vi "Update AppInst Ring.vi"(7 "OpenAppDialog":bool=TRUE, 8 "error in":errorcluster, 9 "Old Value":u16=65535, 10 "AppInst in":refnum<vi>, 11 "Ring in":refnum<vi>) -> (0 "error out":errorcluster, 1 "Selection Changed?":bool, 2 "AppInst out":refnum<vi>)   [LabVIEW 2013, in "LVTM.lvlib"]
uses:
  LVTM.lvlib
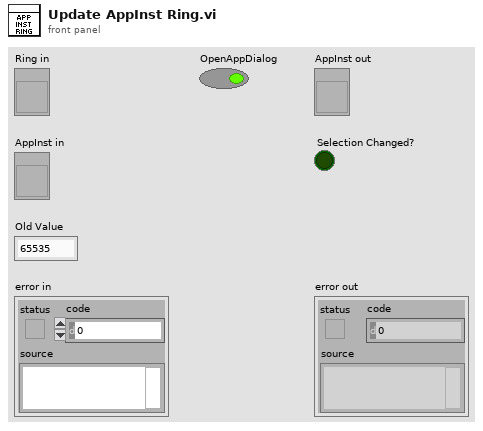
[diagram p1: front panel]
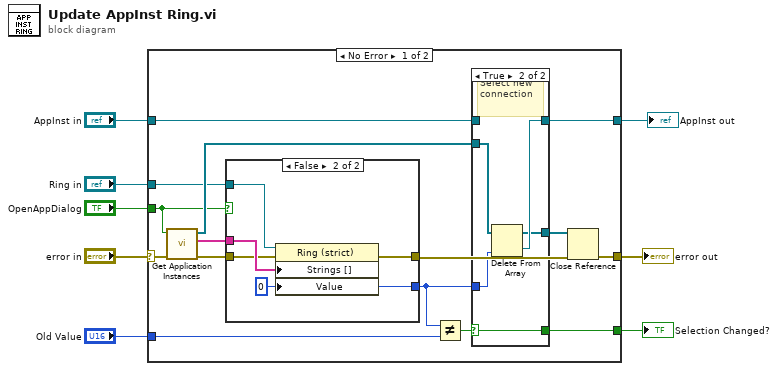
[diagram p0: block diagram]
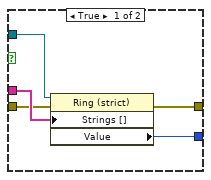
[diagram p2: hidden frame]
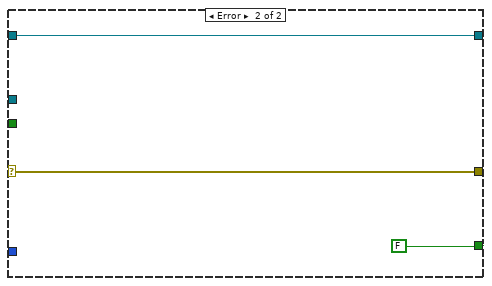
[diagram p4: hidden frame]
diagram:
  n1 = case shown="No Error" "error in" {
    selector: "error in" -> [w19 w44]
    tunnel: "Ring in" -> [w16 _]
    tunnel: [w22 w42] -> w7
    tunnel: "AppInst in" -> [w20 w42]
    tunnel: "Old Value" -> [w12 _]
    tunnel: "OpenAppDialog" -> [w13 _]
    tunnel: [w18 w44] -> w3
    tunnel: [w9 FALSE] -> w2
    frame No Error {
      n2 = call "Get Application Instances.vi"("error in (no error)"=w19, "Update"=w13) -> ("error out"=w15:errorcluster, "App Instance Names"=w17:string[], "App Instances"=w23:refnum<vi>[])  [unwired: 6 in, 1 out]
      n3 = case shown="False" w13 {
        tunnel: w17 -> [w28 w33]
        tunnel: w16 -> [w27 w32]
        tunnel: w15 -> [w26 w31]
        tunnel: [w25 w30] -> w14
        tunnel: [w24 w29] -> w11
        frame True {
          n4 = property class="Ring (strict)"(reference=w27, error in=w26, "Strings []"=w28) -> (error out=w25:errorcluster, "Value"=w24:u16)  [unwired: 1 out]
        }
        frame False {
          w29 = u16 0 ("Value")
          n5 = property class="Ring (strict)"(reference=w32, error in=w31, "Strings []"=w33, "Value"=w29) -> (error out=w30:errorcluster)  [unwired: 1 out]
        }
      }
      n6 = Not Equal?(x=w11, y=w12) -> (x != y?=w10:bool)
      n7 = case shown="True" w10 {
        selector: w10 -> [w34 w37]
        tunnel: w23 -> [w36 w41]
        tunnel: [w35 w40] -> w22
        tunnel: [w36 w39] -> w21
        tunnel: w20 -> [w35 _]
        tunnel: w11 -> [_ w38]
        tunnel: [w34 w37] -> w9
        frame False {
        }
        frame True {
          # "Select new\nconnection"
          n8 = Delete From Array(array=w41, index=w38) -> (deleted portion=w40:refnum<vi>, array with subset deleted=w39:refnum<vi>[])  [unwired: 1 in]
        }
      }
      n9 = Close Reference(reference=w21, error in (no error)=w14) -> (error out=w18:errorcluster)
    }
    frame Error {
    }
  }
  "AppInst out" <- w7
  "Selection Changed?" <- w2
  "error out" <- w3
